vi "Write String Comparator.vi"(8 "error in (no error)":errorcluster, 10 "String Comparator":T1, 11 "String Assertion in":refnum<class "String Assertion.lvclass">) -> (0 "error out":errorcluster, 3 "String Assertion out":refnum<class "String Assertion.lvclass">)   [LabVIEW 2020, in "MacroAssert.lvlib" / "String Assertion.lvclass"]
uses:
  String Assertion.lvclass
  String Comparator.ctl
  String Assertion.lvclass/String Assertion.ctl
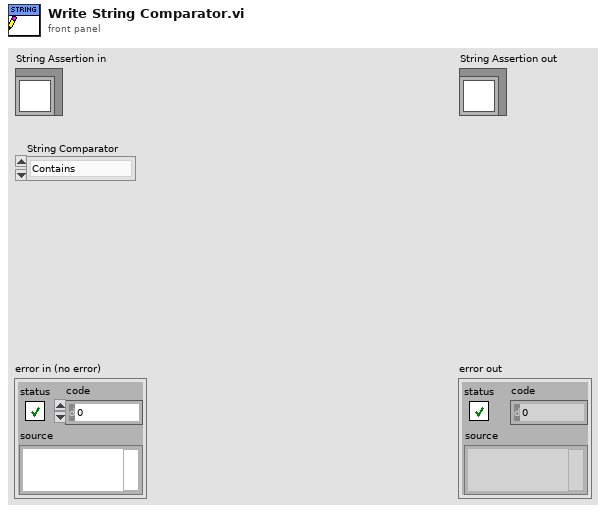
[diagram p1: front panel]
types:
  T1 = typedef "MacroAssert.lvlib/String Assertion.lvclass/String Comparator.ctl" = enum16{"Contains", "Equals", "Starts with", "Ends with", "Does not contain", "Does not equal"}
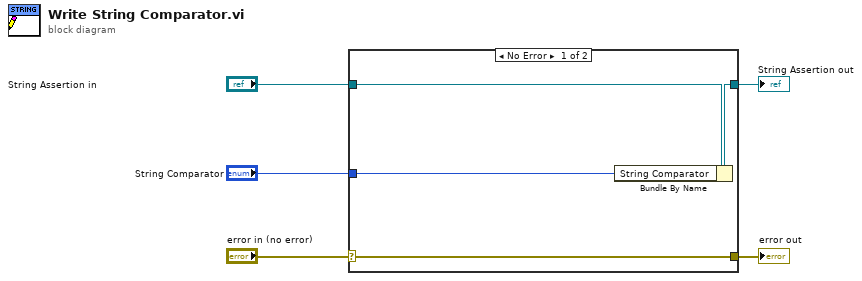
[diagram p0: block diagram]
diagram:
  n1 = case shown="No Error" "error in (no error)" {
    selector: "error in (no error)" -> [w9 w10]
    tunnel: [w9 w10] -> w4
    tunnel: [w7 w11] -> w2
    tunnel: "String Assertion in" -> [w8 w11]
    tunnel: "String Comparator" -> [w6 _]
    frame No Error {
      n2 = Bundle By Name(cluster=w8, "String Comparator"=w6) -> (w7:refnum<class "String Assertion.lvclass">)
    }
    frame Error {
    }
  }
  "error out" <- w4
  "String Assertion out" <- w2
